vi "Read.vi"(8 "error in (no error)":errorcluster caption="entrée d'erreur (pas d'erreur)", 11 "Class CSV_File (Default) en entrée":refnum<class "Class CSV_File.lvclass">) -> (0 "error out":errorcluster caption="sortie d'erreur", 3 "Class CSV_File (Default) en sortie":refnum<class "Class CSV_File.lvclass">)   [LabVIEW 2020, in "Library Instrument & Equipement.lvlib" / "Library File.lvlib" / "Class CSV_File.lvclass"]
doc: "Reads one or more lines depending on the data condition. If the condition is empty, then the line data is taken into account and the function returns the requested line.\nIf the line value is -1, the entire contents of the file will be returned."
uses:
  Class CSV_File.lvclass
  C:/Users/ngarcin/OneDrive - Altyor/Standard TB/Class/Read CSV File/Class File (Default)/Class File (Default).lvclass
  Class File (Default)/Class File (Default).lvclass
  Class CSV_File.lvclass/Class CSV_File.ctl
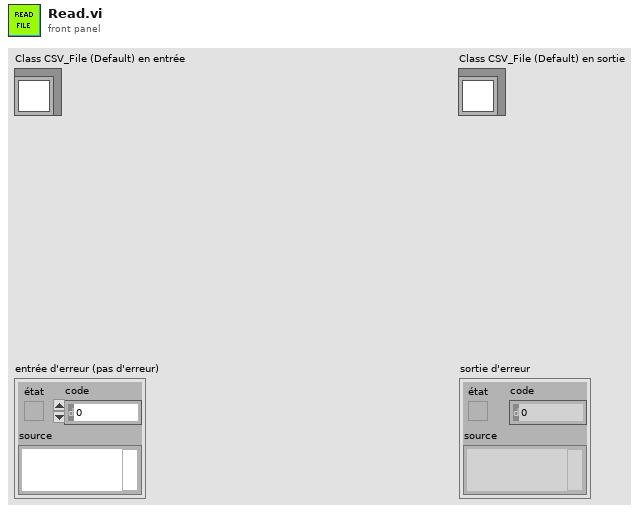
[diagram p1: front panel]
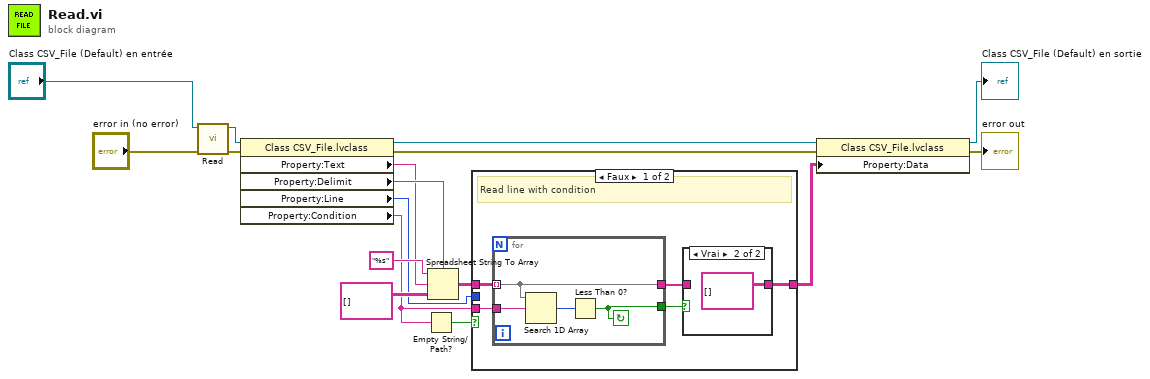
[diagram p0: block diagram]
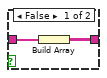
[diagram p2: hidden frame]
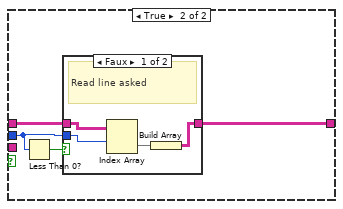
[diagram p3: hidden frame]
diagram:
  n1 = call-parent "Read.vi"("error in (no error)"="error in (no error)", "Class CSV_File (Default) en entrée"="Class CSV_File (Default) en entrée") -> ("error out"=w1:errorcluster, "Class CSV_File (Default) en sortie"=w4:refnum<class "Class CSV_File.lvclass">)  [unwired: 8 in]
  n2 = property class="Class CSV_File.lvclass"(reference=w4, error in=w1) -> (reference out=w13:refnum<class "Class CSV_File.lvclass">, error out=w2:errorcluster, "Property:Text"=w3:string, "Property:Delimit"=w12:string, "Property:Line"=w7:i16, "Property:Condition"=w5:string)
  n3 = Empty String/Path?(string/path=w5) -> (empty?=w11:bool)
  n4 = Spreadsheet String To Array(delimiter (Tab)=w12, format string="%s" ("chaîne de format"), spreadsheet string=w3, array type (2D Dbl)=string[][] [] ("type (empty)")) -> (array=w8:string[][])
  n5 = case shown="Faux" w11 {
    tunnel: w8 -> [w22 w31]
    tunnel: w7 -> [_ w30]
    tunnel: [w19 w32] -> w6
    tunnel: w5 -> [w21 _]
    frame False {
      # "Read line with condition"
      n6 = for {
        tunnel: w22 -> [w27] mode=indexing
        tunnel: w21 -> [w29]
        tunnel: [w27] -> w20
        tunnel: [w26] -> w18
        stop <- w26 continue-if-true
        n7 = Search 1D Array(1D array=w27, element=w29) -> (index of element=w28:i32)  [unwired: 1 in]
        n8 = Less Than 0?(x=w28) -> (x < 0?=w26:bool)
      }
      n9 = case shown="Vrai" w18 {
        tunnel: w20 -> [w24 _]
        tunnel: [w23 string[][] []] -> w19
        frame False {
          n10 = Build Array(w24) -> (w23:string[][])
        }
        frame True {
        }
      }
    }
    frame True {
      n11 = Less Than 0?(x=w30) -> (x < 0?=w33:bool)
      n12 = case shown="Faux" w33 {
        tunnel: [w35 w38] -> w32
        tunnel: w31 -> [w37 w38]
        tunnel: w30 -> [w34 _]
        frame False {
          # "Read line asked"
          n13 = Index Array(array=w37, index (row)=w34) -> (element=w36:string[])  [unwired: 1 in]
          n14 = Build Array(w36) -> (w35:string[][])
        }
        frame True {
          # "If line <0 read All"
        }
      }
    }
  }
  n15 = property class="Class CSV_File.lvclass"(reference=w13, error in=w2, "Property:Data"=w6) -> (reference out=→"Class CSV_File (Default) en sortie":refnum<class "Class CSV_File.lvclass">, error out=→"error out":errorcluster)
